vi "JSON TO current.vi"(7 "IP":string="192.168.23.100", 8 "error in (no error)":errorcluster, 10 "PORT":dbl=1.0 min=1.0 max=4.0 step=1.0, 11 "MASTER":dbl=1.0 min=1.0 max=10.0 step=1.0) -> (0 "error out":errorcluster, 3 "CURRENT":u32 format="%.0f mA")   [LabVIEW 2024]
uses:
  <vilib>/JDP Science/JSONtext/JSONtext.lvlib
  <userlib>/_OpenG.lib/string/string.llb/openg_string.lvlib
panel:
  out "JSON data":string
  # "Smart conn. current data"
  # "Only 100% duty cycle!!"
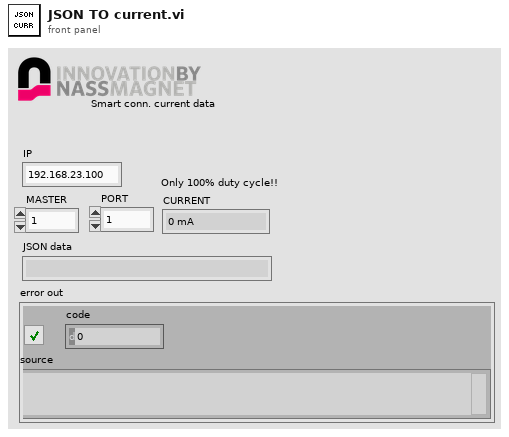
[diagram p1: front panel]
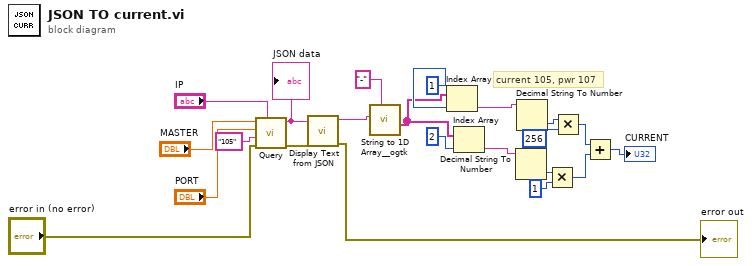
[diagram p0: block diagram]
diagram:
  # "current 105, pwr 107"
  n1 = call "Query.vi"("IP"="IP", "error in (no error)"="error in (no error)", "PARAMETERS"="105", "PORT"="PORT", "MASTER"="MASTER") -> ("error out"=w14:errorcluster, "JSON data"=w22:string)  [unwired: 5 in]
  "JSON data" <- w22
  n2 = call <vilib>:"Display Text from JSON.vi"("error in (no error)"=w14, "Input JSON"=w22) -> ("error out"=→"error out":errorcluster, "Display Text"=w9:string)  [unwired: 7 in, 1 out]
  n3 = call <userlib>:"String to 1D Array__ogtk.vi"("delimiter (Tab)"="-", "string"=w9) -> ("Array of Strings"=w1:string[])  [unwired: 9 in]
  n4 = Index Array(array=w1, index=1) -> (element=w2:string)
  n5 = Index Array(array=w1, index=2) -> (element=w3:string)
  n6 = Decimal String To Number(string=w3) -> (number=w11:i32)  [unwired: 2 in, 1 out]
  n7 = Decimal String To Number(string=w2) -> (number=w7:i32)  [unwired: 2 in, 1 out]
  n8 = Multiply(x=w11, y=u32 1) -> (x*y=w10:u32)
  n9 = Multiply(x=w7, y=u32 256) -> (x*y=w8:u32)
  n10 = Add(x=w8, y=w10) -> (x+y=→"CURRENT":u32)
